vi "Export time-speed data subset.vi"(7 "Funct data structure":bool, 8 "error in (no error)":errorcluster, 10 "Existing AVI path":path, 11 "New folder path":path) -> (0 "error out":errorcluster, 4 "Extraction cursors":cluster{"Min cursor":i32, "Max cursor":i32}, 6 "# of Frames in exported portion":i32)   [LabVIEW 2020]
uses:
  Globals/gl_Time series viewer globals.vi
  <userlib>/My Palettes.lib/Files & paths/Spreadsheet/Write To Spreadsheet File (string)-Mod.vi
panel:
  out "Valid speed data array size":i32[](array[numeric])
  out "Number of speed points/rows":dbl
  out "Size of extracted speed data portion":i32[](array[numeric])
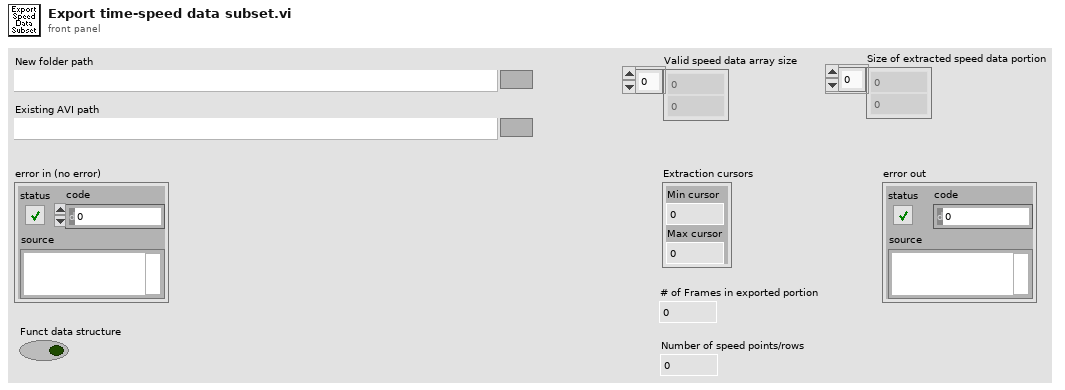
[diagram p1: front panel]
types:
  T1 = typedef "Time series viewer refs.ctl" = cluster{"This VI":refnum<vi>, "Image control":refnum<vi>, "AVI Mode ind":refnum<vi>, "Play":refnum<vi>, "Stop":refnum<vi>, "Back":refnum<vi>, "Scrollbar":refnum<vi>, "Video length info":refnum<vi>, "Expected speed values":refnum<vi>, "Intensity":refnum<vi>, "Path":refnum<vi>, "Selection sliders":refnum<vi>, "Speed Graph ref":refnum<vi>, "Frame rate set (fps)":refnum<vi>, "Number of rows to generate":refnum<vi>, "VL Image Array":refnum<vi>, "Image Scrollbar":refnum<vi>, "Channel to load":refnum<vi>, "Colour":refnum<vi>}
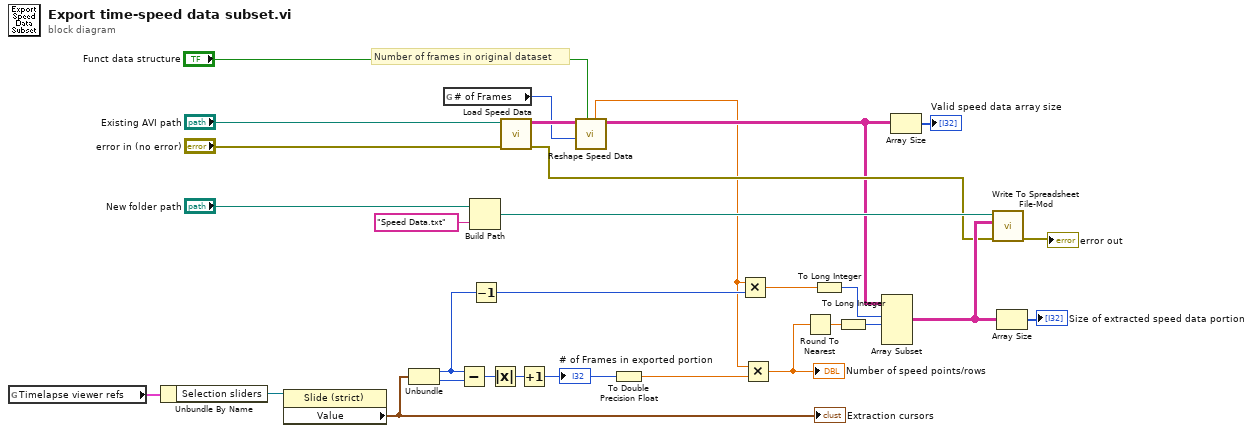
[diagram p0: block diagram]
diagram:
  # "Number of frames in original dataset"
  n1 = global read "gl_Time series viewer globals.vi" "Timelapse viewer refs"() -> (w12:T1)
  n2 = Unbundle By Name(w12) -> ("Selection sliders"=w13:refnum<vi>)
  n3 = property class="Slide (strict)"(reference=w13) -> ("Value"=w3:cluster{i32, i32})  [unwired: 1 in, 2 out]
  "Extraction cursors" <- w3
  n4 = Unbundle(w3) -> (w2:i32, w11:i32)
  n5 = global read "gl_Time series viewer globals.vi" "# of Frames"() -> (w18:u32)
  n6 = Subtract(x=w2, y=w11) -> (x-y=w10:i32)
  n7 = Build Path(base path="New folder path", name or relative path="Speed Data.txt") -> (appended path=w29:path)
  n8 = Decrement(x=w2) -> (x-1=w16:i32)
  n9 = Absolute Value(x=w10) -> (abs(x)=w9:i32)
  n10 = call "Load Speed Data.vi"("error in (no error)"="error in (no error)", "AVI File Path"="Existing AVI path") -> ("error out"=w21:errorcluster, "Speed Data"=w23:string[][])  [unwired: 8 in]
  n11 = Increment(x=w9) -> (x+1=w4:i32)
  "# of Frames in exported portion" <- w4
  n12 = call "Reshape Speed Data.vi"("Funct data structure"="Funct data structure", "Number of time series microscope data frames"=w18, "all rows"=w23) -> ("Speed Data"=w20:string[][], "Points per frame (fractional)"=w8:dbl)  [unwired: 3 in, 4 out]
  n13 = To Double Precision Float(number=w4) -> (double precision float=w7:dbl)
  n14 = Multiply(x=w8, y=w16) -> (x*y=w15:dbl)
  n15 = Multiply(x=w8, y=w7) -> (x*y=w6:dbl)
  "Number of speed points/rows" <- w6
  n16 = Round To Nearest(number=w6) -> (nearest integer value=w17:dbl)
  n17 = To Long Integer(number=w15) -> (32bit integer=w5:i32)
  n18 = To Long Integer(number=w17) -> (32bit integer=w14:i32)
  n19 = Array Subset "Array Subset"(array=w20, index (row)=w5, length (row)=w14) -> (w26:string[][])  [unwired: 2 in]
  n20 = Array Size(array=w20) -> (size(s)=→"Valid speed data array size":i32[])
  n21 = call-poly <userlib>:"Write To Spreadsheet File-Mod.vi"("error in"=w21, "2D data"=w26, "file path (dialog if empty)"=w29) -> ("error out"=→"error out":errorcluster)  [unwired: 7 in, 1 out]
  n22 = Array Size(array=w26) -> (size(s)=→"Size of extracted speed data portion":i32[])
